vi "Get Pixel by Pollling(DEMO).vi"() -> ()   [LabVIEW 2011]
panel:
  in  "停止按钮":bool
  out "Color":u32(colorbox)
  out "Load Picture":picture caption="载入图片"
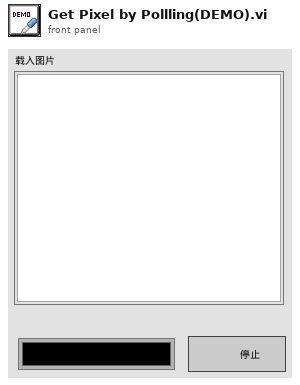
[diagram p1: front panel]
types:
  T1 = typedef "imagedata.ctl" = cluster{"image type":i32, "image depth":i32, "image":u8[], "mask":u8[], "colors":u32[], "Rectangle":cluster{"left":i16, "top":i16, "right":i16, "bottom":i16}}
  T2 = typedef "LVMouseTypeDef.ctl" = cluster{"Mouse Position":cluster{"X":i32, "Y":i32}, "Mouse Modifiers":cluster{"Button Down":bool, "Shift Mod":bool, "Menu Mod":bool, "Option Mod":bool}}
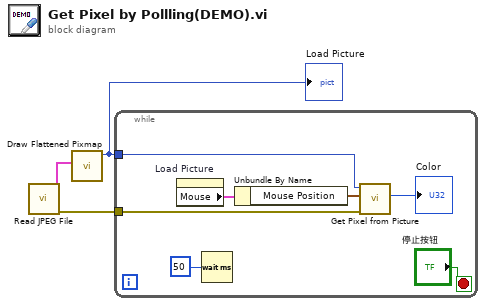
[diagram p0: block diagram]
diagram:
  n1 = call <vilib>:"Read JPEG File.vi"() -> ("error out"=w1:errorcluster, "image data"=w3:T1)  [unwired: 9 in, 1 out]
  n2 = call <vilib>:"Draw Flattened Pixmap.vi"("image data"=w3) -> ("new picture"=w2:picture)  [unwired: 8 in]
  "Load Picture" <- w2
  n3 = while {
    tunnel: w2 -> [w7]
    tunnel: w1 -> [w10]
    stop <- "停止按钮" stop-if-true
    n4 = property on="Load Picture" class="Pict"() -> ("Mouse"=w9:T2)  [unwired: 2 in, 2 out]
    n5 = Wait (ms)(milliseconds to wait=u32 50 ("等待时间（毫秒）")) -> ()  [unwired: 1 out]
    n6 = Unbundle By Name(w9) -> ("Mouse Position"=w8:cluster{"X":i32, "Y":i32})
    n7 = call "Get Pixel from Picture.vi"("错误输入"=w10, "Pos"=w8, "Picture in"=w7) -> ("Color"=→"Color":u32)  [unwired: 6 in, 2 out]
  }
